vi "is_roi_empty.vi"(1 "ROI":T1) -> (0 "roi empty":bool)   [LabVIEW 2018]
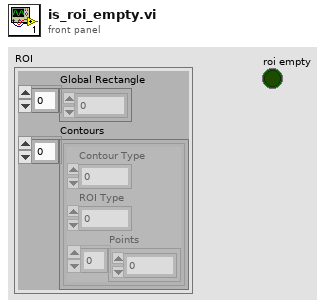
[diagram p1: front panel]
types:
  T1 = cluster{"Global Rectangle":i32[], "Contours":cluster{"Contour Type":u32, "ROI Type":u32, "Points":i32[]}[]}
  T2 = cluster{"Contour Type":u32, "ROI Type":u32, "Points":i32[]}[]
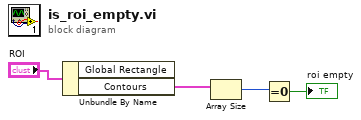
[diagram p0: block diagram]
diagram:
  n1 = Unbundle By Name("ROI") -> ("Contours"=w3:T2)  [unwired: 1 out]
  n2 = Array Size(array=w3) -> (size(s)=w2:i32)
  n3 = Equal To 0?(x=w2) -> (x = 0?=→"roi empty":bool)
